vi "Destroy User Event - Stop.vi"(0 "Stop Event Registeration":refnum<event-registration> caption="事件注册引用句柄", 1 "User Event - Stop":refnum<user-event> caption="用户事件－停止", 3 "error in (no error)":errorcluster caption="错误输入（无错误）") -> (10 "error out":errorcluster caption="错误输出")   [LabVIEW 2013, in "User Event - Stop.lvlib"]
doc: "无论是否即将出错，销毁用户事件。"
uses:
  User Event - Stop.lvlib
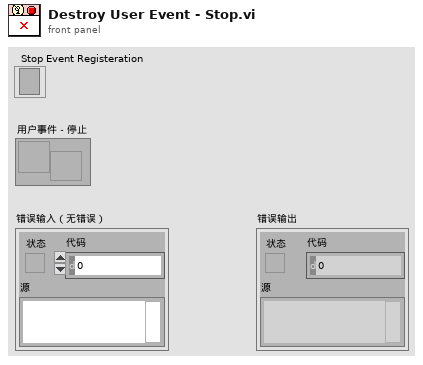
[diagram p1: front panel]
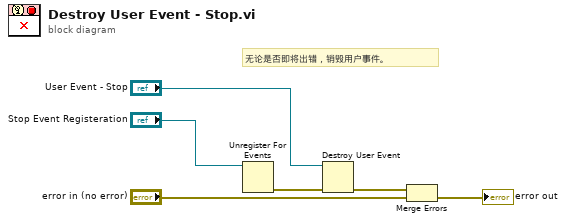
[diagram p0: block diagram]
diagram:
  # "无论是否即将出错，销毁用户事件。"
  n1 = Unregister For Events(event registration refnum="Stop Event Registeration") -> (error out=w6:errorcluster)  [unwired: 1 in]
  n2 = Destroy User Event(user event="User Event - Stop", error in=w6) -> (error out=w4:errorcluster)
  n3 = Merge Errors(w4, "error in (no error)") -> (→"error out":errorcluster)
